vi "主界面.vi"() -> ()   [LabVIEW 2010]
uses:
  全局量/全局_配置.vi
  全局量/试验配置信息.vi
  全局量/自动测试结果.vi
panel:
  in  "?":enum32{"测试类型 1", "测试类型 2"}(tab)
  in  "单选_数字量输入":bool
  in  "单选_数字量输出":bool
  in  "单选_DSP输入":bool
  in  "单选_CAN检测":bool
  in  "单选_LAN检测":bool
  in  "单选_R232检测":bool
  in  "btn_数字输出":bool
  in  "btn_DSP输入":bool
  in  "btn_CAN总线":bool
  in  "btn_LAN总线":bool
  in  "btn_R232总线":bool
  in  "btn_开始检测":bool
  in  "btn_数字输入":bool
  in  "btn_R485总线":bool
  out "进度":u8(slide) scale=0.0..100.0
  in  "单选_R485检测":bool
  in  "单选_AD输入":bool
  out "数字量输入检测":bool
  out "数字量输出检测":bool
  out "模拟量DSP输入检测":bool
  out "模拟量AD输入检测":bool
  out "CAN总线检测":bool
  out "LAN总线检测":bool
  out "RS232总线检测":bool
  out "RS485总线检测":bool
  in  "函数类型 4":bool
  in  "通道及参数配置":bool
  in  "函数类型 2":bool
  in  "函数类型 3":bool
  in  "函数类型 1":bool
  in  "进度每次增加数":dbl
  in  "电路板类型":T1(ring)
  in  "btn_二维码识别":bool
  out "退出？":bool
  in  "btn_退出":bool
  out "时间标识":timestamp format="%<%H:%M:%S>T"
  in  "btn_报告管理":bool
  in  "btn_生成报表":bool
  in  "btn_保存结果":bool
  in  "str_测试地点":string
  in  "str_测试人员":string
  in  "str_测试编号":string
  in  "str_报告编号":string
  out "检测信息":string[][](table)
  in  "btn_控制板配置":bool
  # "TNB-S600KZ型控制板自动化检测装置"
  # "测试报告信息"
  # "板 卡 试  验  信  息"
  # "试验报告编号："
  # "测试板卡编号："
  # "板卡类型："
  # "测试人员："
  # "测试地点："
  # "系统时间:"
  # "自动检测"
  # "分步检测"
  # "检\n测\n项\n目"
  # "检测进度"
  # "配置选项"
  # "分步检测"
  # "检\n测\n项\n目"
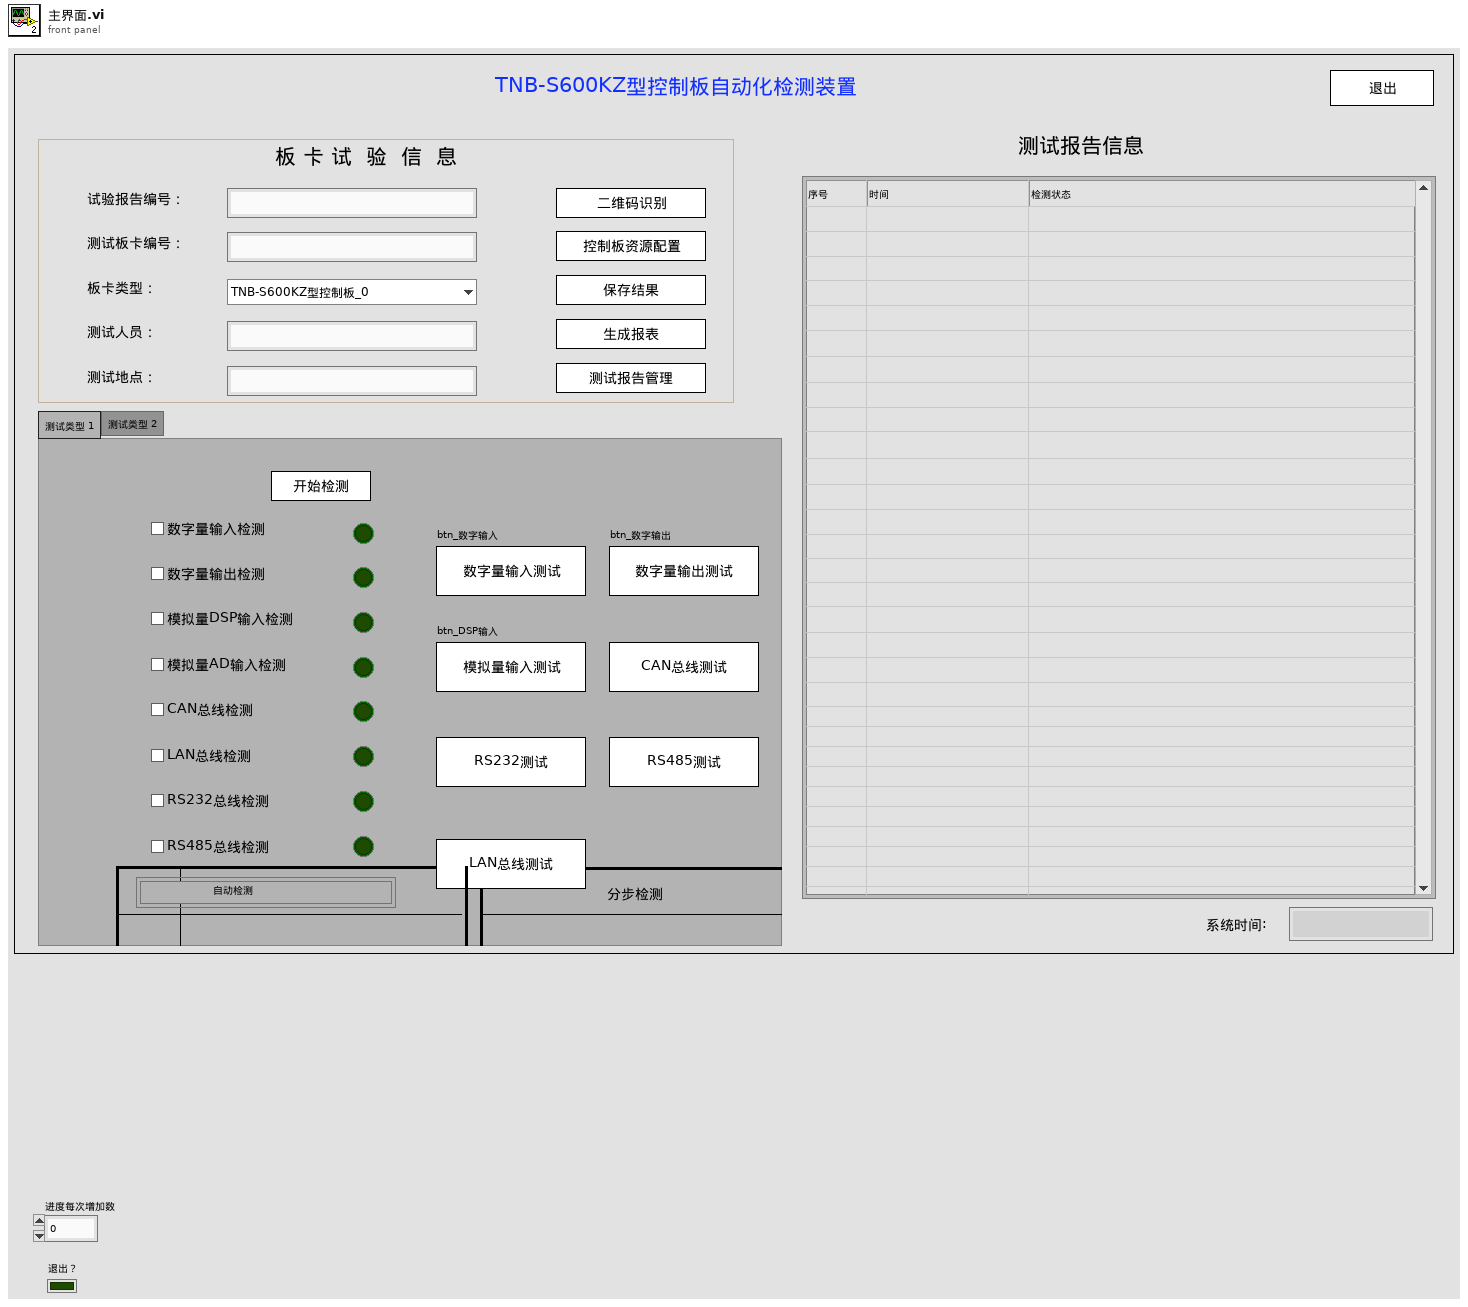
[diagram p1: front panel]
types:
  T1 = enum16{"TNB-S600KZ型控制板_0", "TNB-S600KZ型控制板_1", "TNB-S600KZ型控制板_2"}
  T2 = cluster{"数字量输入信号路数":u32, "数字量输出信号路数":u32, "DSP模拟量输入信号路数":u32, "DSP模拟量输入信号幅值":u32, "AD模拟量输入信号路数":u32, "AD模拟量输入信号幅值":u32, "RS232端口":u32, "RS232通信路数":u32, "RS232波特率":u32, "RS485端口":u32, "RS485通信路数":u32, "RS485波特率":u32, "CAN通信端口":string, "CAN波特率":u32, "以太网选择?":bool, "控制板IP":string, "以太网端口":u32}
  T3 = cluster{"str_报告编号":string, "str_测试板卡编号":string, "str_测试人员":string, "str_测试地点":string, "str_测试板卡类型":string}
  T4 = cluster{"str_报告编号":string, "str_测试编号":string, "str_测试人员":string, "str_测试地点":string, string}
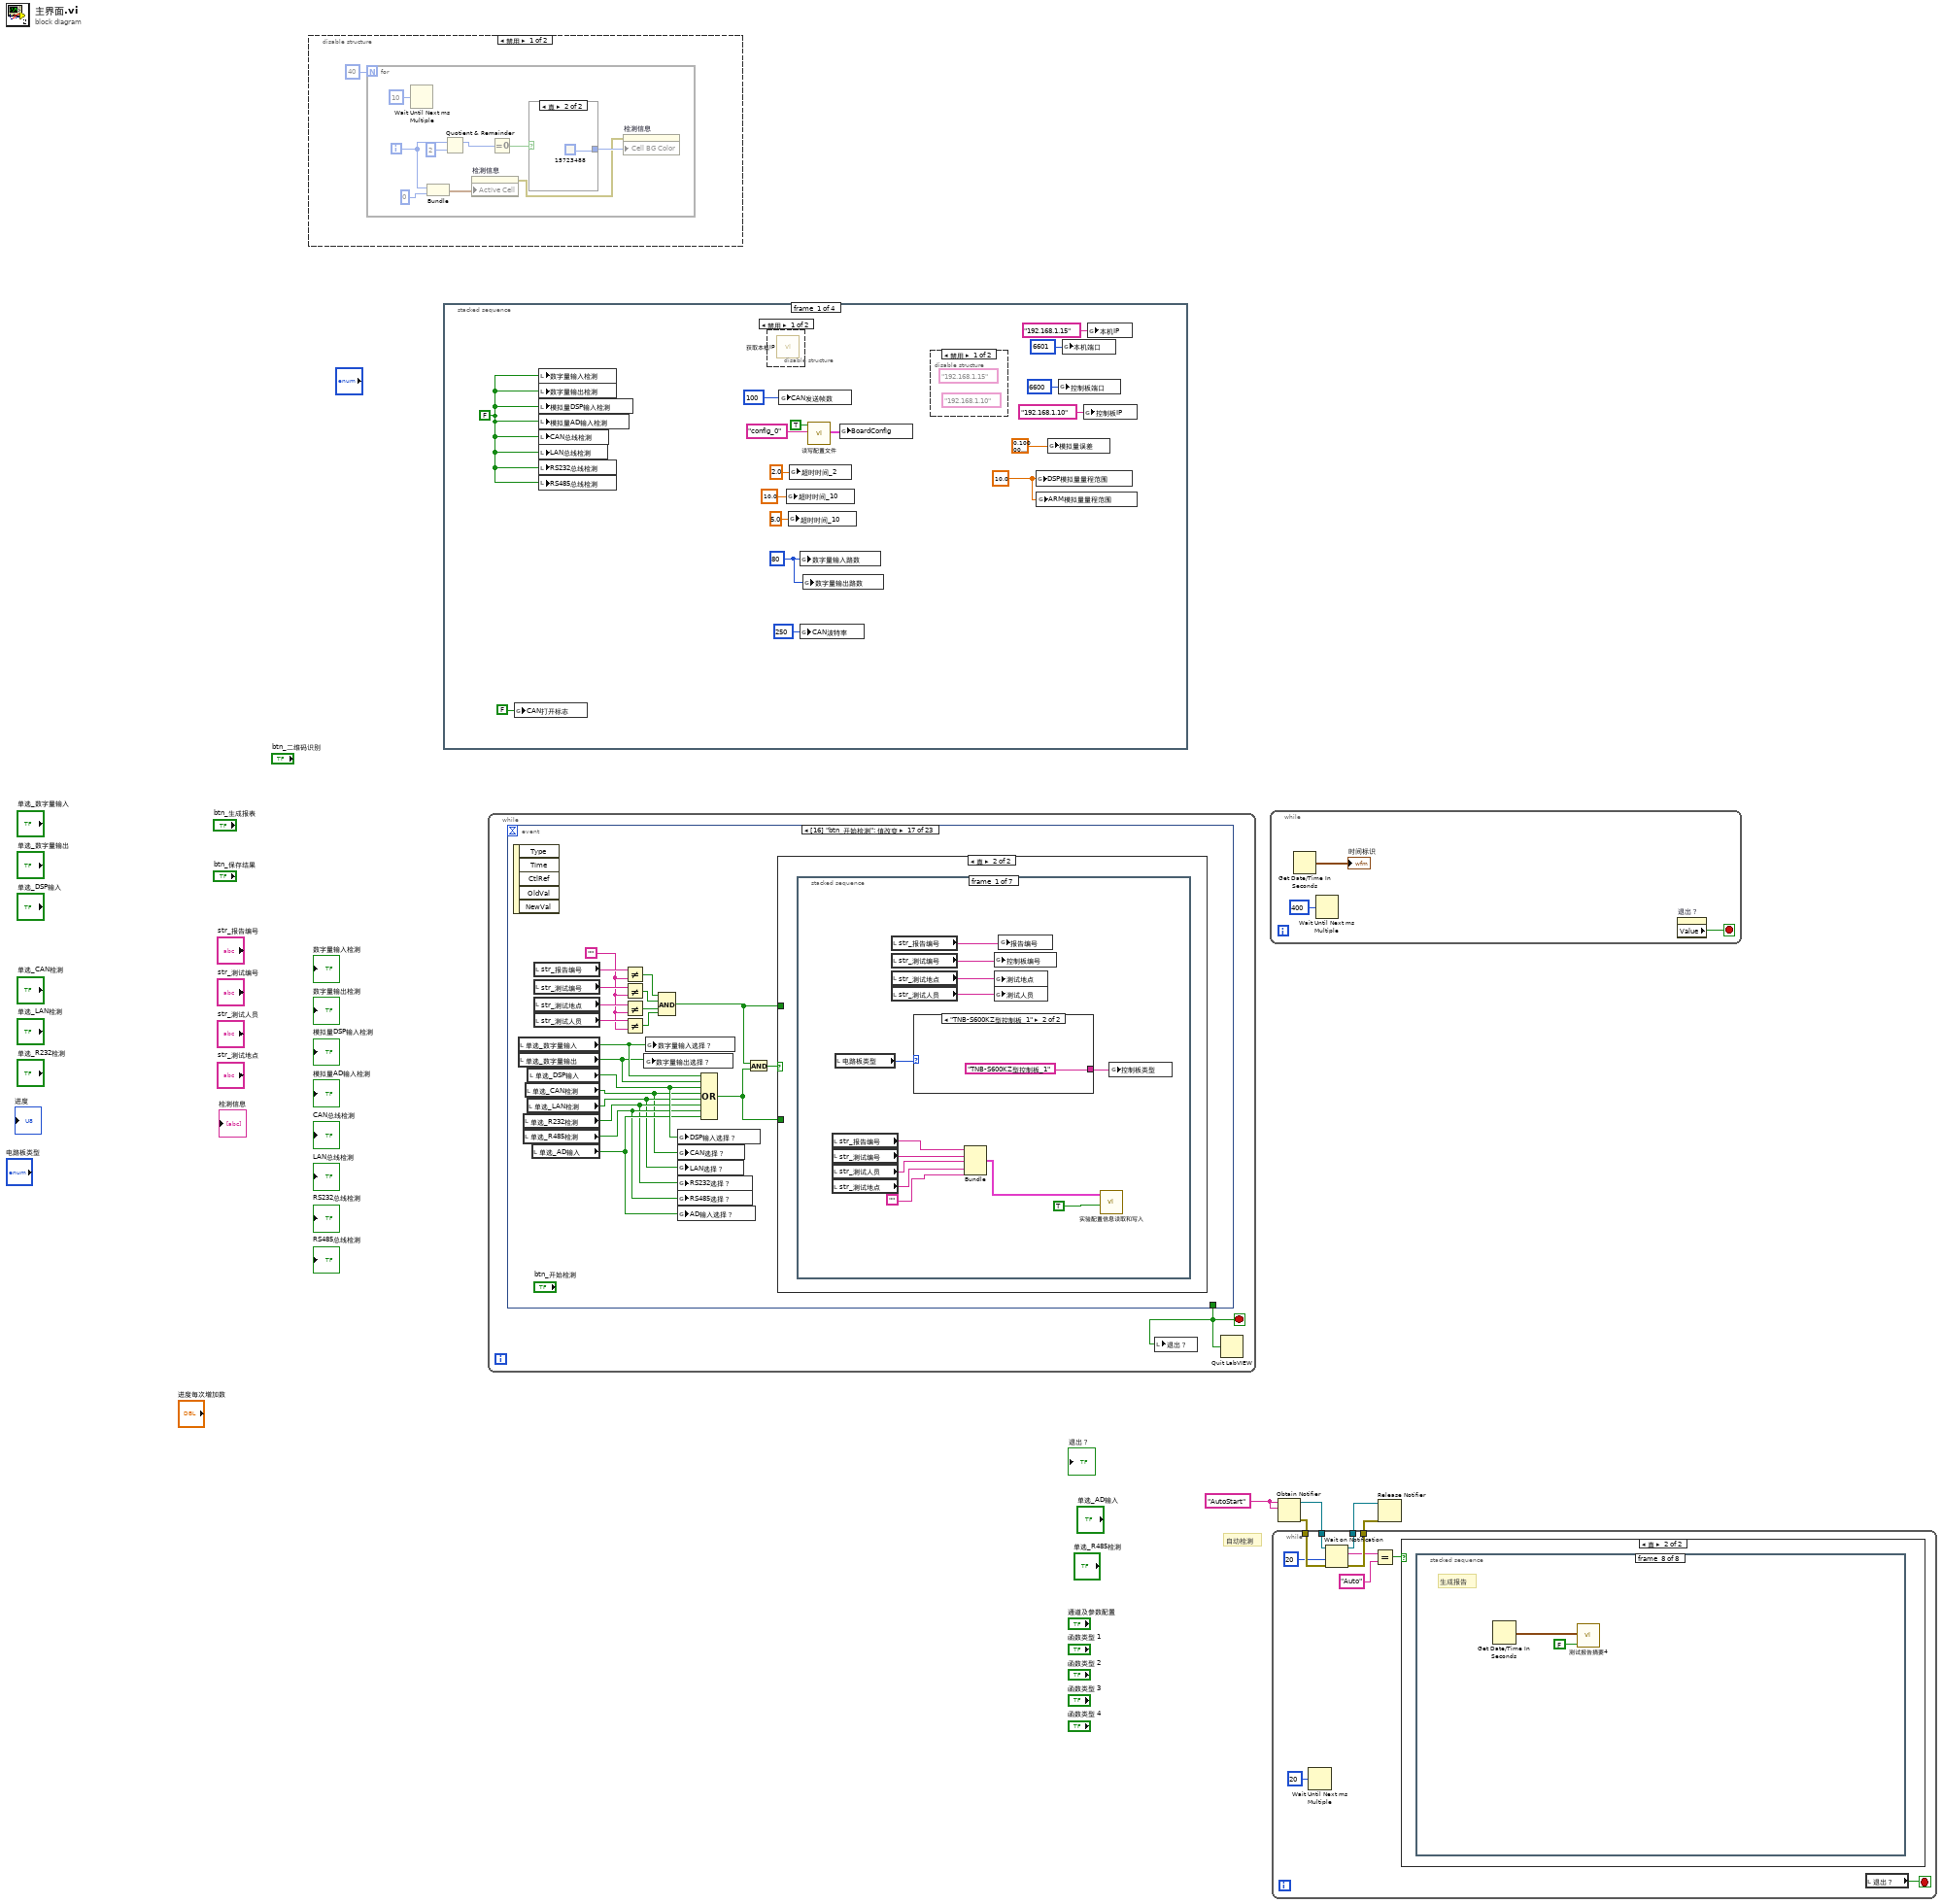
[diagram p0: block diagram]
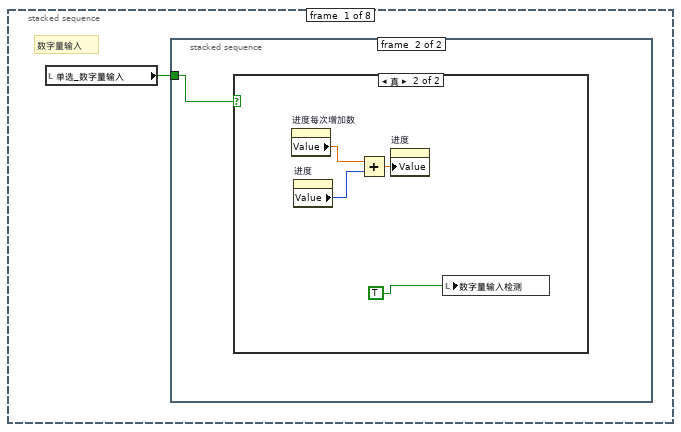
[diagram p3: hidden frame]
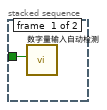
[diagram p4: hidden frame]
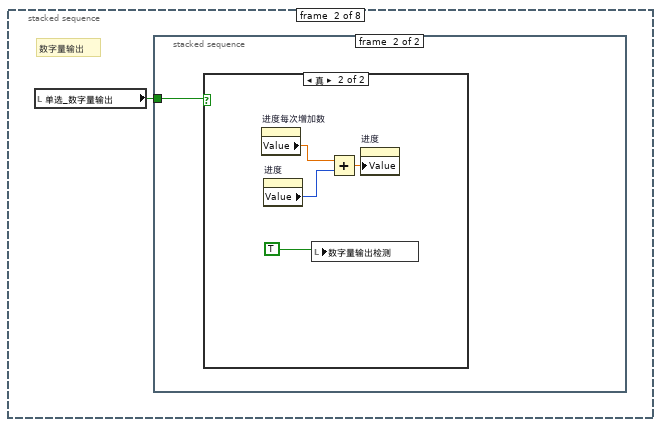
[diagram p6: hidden frame]
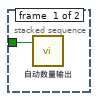
[diagram p7: hidden frame]
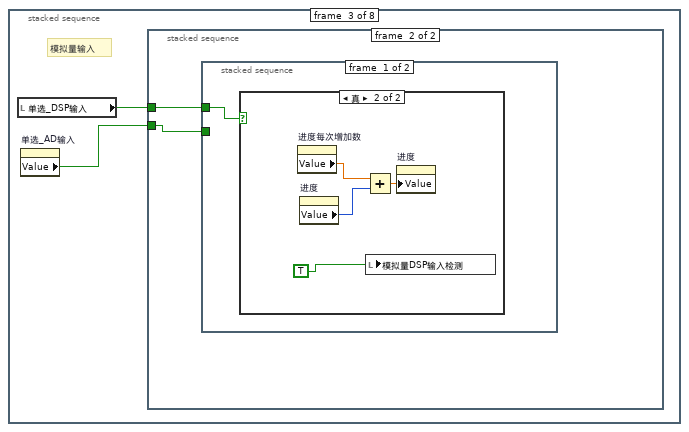
[diagram p9: hidden frame]
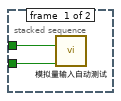
[diagram p10: hidden frame]
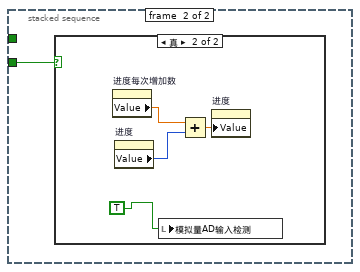
[diagram p12: hidden frame]
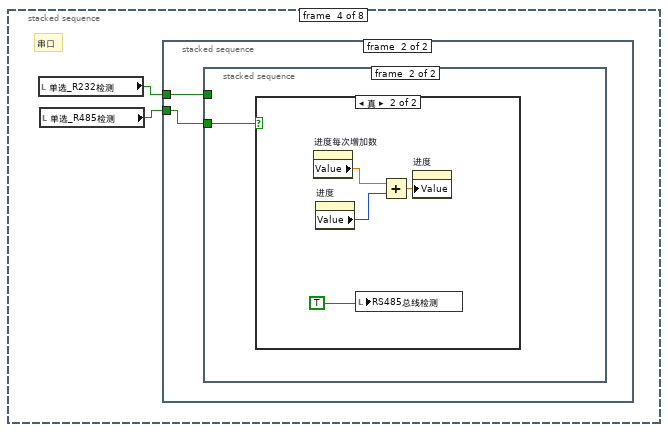
[diagram p14: hidden frame]
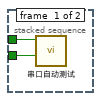
[diagram p15: hidden frame]
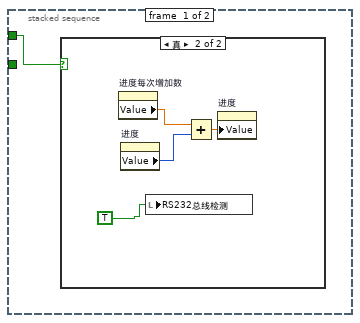
[diagram p16: hidden frame]
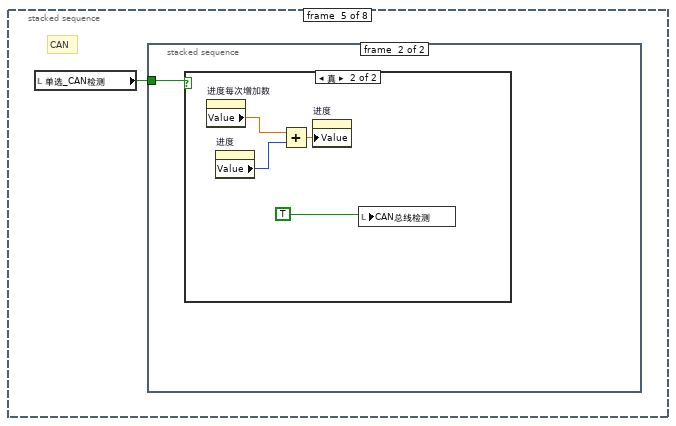
[diagram p19: hidden frame]
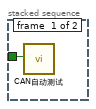
[diagram p20: hidden frame]
diagram:
  w5 = "AutoStart" ("名称（未命名）")
  # "自动检测"
  n1 = disable-structure shown="禁用" {
    frame Disabled {
      n2 = for {
        N: 40 -> [_]
        i -> [w10]
        n3 = Wait Until Next ms Multiple(millisecond multiple=u32 10 ("毫秒倍数")) -> ()  [unwired: 1 out]
        n4 = Bundle(w10, 0) -> (w11:cluster{i32, i32})  [unwired: 1 in]
        n5 = Quotient & Remainder(x=w10, y=2) -> (x-y*floor(x/y)=w8:i32)  [unwired: 1 out]
        n6 = property on="检测信息" class="Tbl (严格)"("Active Cell"=w11) -> (error out=w7:errorcluster)  [unwired: 2 in, 1 out]
        n7 = Equal To 0?(x=w8) -> (x = 0?=w15:bool)
        n8 = case shown="真" w15 {
          tunnel: [u32 16448250 u32 15723488] -> w14
          frame False {
          }
          frame True {
          }
        }
        n9 = property on="检测信息" class="Tbl (严格)"(error in=w7, "Cell BG Color"=w14) -> ()  [unwired: 1 in, 2 out]
      }
    }
    frame Enabled {
    }
  }
  n10 = stacked-sequence {
    frame #0 {
      w18 = FALSE
      w20 = 80 ("数字量输入路数")
      w21 = sgl 10.0 ("DSP模拟量量程范围")
      n11 = global write "全局_配置.vi" "CAN打开标志"(FALSE ("CAN打开标志")) -> ()
      n12 = local write "数字量输入检测"(w18) -> ()
      n13 = local write "数字量输出检测"(w18) -> ()
      n14 = local write "模拟量DSP输入检测"(w18) -> ()
      n15 = local write "模拟量AD输入检测"(w18) -> ()
      n16 = local write "CAN总线检测"(w18) -> ()
      n17 = local write "LAN总线检测"(w18) -> ()
      n18 = local write "RS232总线检测"(w18) -> ()
      n19 = local write "RS485总线检测"(w18) -> ()
      n20 = disable-structure shown="禁用" {
        frame Disabled {
          n21 = call "获取本机IP.vi"() -> ()  [unwired: 9 in, 3 out]
        }
        frame Enabled {
        }
      }
      n22 = global write "全局_配置.vi" "CAN发送帧数"(u32 100 ("CAN发送帧数")) -> ()
      n23 = global write "全局_配置.vi" "超时时间_10"(10.0 ("超时时间_102")) -> ()
      n24 = global write "全局_配置.vi" "超时时间_10"(5.0 ("超时时间_10")) -> ()
      n25 = global write "全局_配置.vi" "超时时间_2"(2.0 ("超时时间_2")) -> ()
      n26 = global write "全局_配置.vi" "数字量输入路数"(w20) -> ()
      n27 = global write "全局_配置.vi" "CAN波特率"(u16 250 ("CAN波特率")) -> ()
      n28 = global write "全局_配置.vi" "数字量输出路数"(w20) -> ()
      n29 = call "读写配置文件.vi"("文件名称"="config_0", "m_bRead"=TRUE) -> ("BoardConfig_output"=w32:T2)  [unwired: 9 in]
      n30 = global write "全局_配置.vi" "BoardConfig"(w32) -> ()
      n31 = disable-structure shown="禁用" {
        frame Disabled {
          (unwired) "192.168.1.15" ("本机IP")
          (unwired) "192.168.1.10" ("控制板IP")
        }
        frame Enabled {
        }
      }
      n32 = global write "全局_配置.vi" "DSP模拟量量程范围"(w21) -> ()
      n33 = global write "全局_配置.vi" "ARM模拟量量程范围"(w21) -> ()
      n34 = global write "全局_配置.vi" "模拟量误差"(sgl 0.1 ("模拟量误差")) -> ()
      n35 = global write "全局_配置.vi" "控制板端口"(u16 6600 ("控制板端口")) -> ()
      n36 = global write "全局_配置.vi" "本机端口"(u16 6601 ("本机端口")) -> ()
      n37 = global write "全局_配置.vi" "控制板IP"("192.168.1.10" ("控制板IP")) -> ()
      n38 = global write "全局_配置.vi" "本机IP"("192.168.1.15" ("本机IP")) -> ()
    }
    frame #1 {
      w41 = 16 ("维数大小")
      n39 = global write "试验配置信息.vi" "自测DO路数"(76 ("自测DO路数")) -> ()
      n40 = global write "试验配置信息.vi" "自测DI路数"(80 ("自测DI路数")) -> ()
      n41 = global write "试验配置信息.vi" "自测RS232路数"(2 ("自测RS232路数")) -> ()
      n42 = global write "试验配置信息.vi" "自测485路数"(1 ("自测485路数")) -> ()
      n43 = global write "试验配置信息.vi" "自测CAN路数"(4 ("自测CAN路数")) -> ()
      n44 = global write "试验配置信息.vi" "自测LAN路数"(1 ("自测LAN路数")) -> ()
      n45 = global write "试验配置信息.vi" "自测AI_DSP路数"(w41) -> ()
      n46 = global write "试验配置信息.vi" "自测AI_AD路数"(w41) -> ()
    }
    frame #2 {
      w58 = TRUE ("单选_数字量输入")
      # "自动测试"
      n47 = global write "自动测试结果.vi" "DI自动测试结果"(string[][] [["序号", "检测内容", "结果"]] ("自动测试结果")) -> ()
      n48 = local write "str_报告编号"("B001001000001" ("通知")) -> ()
      n49 = local write "str_测试地点"("1号实验室" ("str_测试地点")) -> ()
      n50 = global read "试验配置信息.vi" "自测AI_DSP路数"() -> (w54:i32)
      n51 = global read "试验配置信息.vi" "自测RS232路数"() -> (w43:i32)
      n52 = global read "试验配置信息.vi" "自测AI_AD路数"() -> (w53:i32)
      n53 = global read "试验配置信息.vi" "自测CAN路数"() -> (w49:i32)
      n54 = global read "试验配置信息.vi" "自测485路数"() -> (w46:i32)
      n55 = Initialize Array(TRUE ("元素"), w49) -> (w48:bool[])
      n56 = Initialize Array(TRUE ("元素"), w46) -> (w47:bool[])
      n57 = local write "单选_数字量输入"(w58) -> ()
      n58 = local write "单选_数字量输出"(w58) -> ()
      n59 = local write "单选_DSP输入"(w58) -> ()
      n60 = local write "单选_CAN检测"(w58) -> ()
      n61 = local write "单选_LAN检测"(w58) -> ()
      n62 = local write "单选_R232检测"(w58) -> ()
      n63 = local write "单选_R485检测"(w58) -> ()
      n64 = local write "单选_AD输入"(w58) -> ()
      n65 = Initialize Array(TRUE ("元素"), w54) -> (w59:bool[])
      n66 = Initialize Array(TRUE ("元素"), w43) -> (w42:bool[])
      n67 = Initialize Array(TRUE ("元素"), w53) -> (w51:bool[])
      n68 = global write "自动测试结果.vi" "Auto_RS485_R"(w47) -> ()
      n69 = global write "自动测试结果.vi" "Auto_RS232_R"(w42) -> ()
      n70 = global write "自动测试结果.vi" "Auto_CAN_R"(w48) -> ()
      n71 = global write "自动测试结果.vi" "Auto_DSP_R"(w59) -> ()
      n72 = global write "自动测试结果.vi" "Auto_AD_R"(w51) -> ()
      n73 = property on="进度" class="Slide (严格)"("Value"=u8 0 ("进度")) -> ()  [unwired: 2 in, 2 out]
      n74 = global write "试验配置信息.vi" "自测类数"(0 ("自动测试个数")) -> ()
    }
    frame #3 {
      n75 = call "实验配置信息读取和写入.vi"("读取写入"=FALSE) -> ("簇 2"=w67:T3)  [unwired: 10 in]
      n76 = Unbundle By Name(w67) -> ("str_报告编号"=w66:string, "str_测试板卡编号"=w65:string, "str_测试人员"=w64:string, "str_测试地点"=w63:string)  [unwired: 1 out]
      n77 = local write "str_报告编号"(w66) -> ()
      n78 = local write "str_测试编号"(w65) -> ()
      n79 = local write "str_测试人员"(w64) -> ()
      n80 = local write "str_测试地点"(w63) -> ()
    }
  }
  n81 = while {
    stop <- w69 stop-if-true
    n82 = event shown="[16] \"btn_开始检测\": 值改变" {
      selector: _ -> [_ _ _ _ _ _ _ _ _ _ _ _ _ _ _ _ _ _ _ _ _ _ _]
      dyn-events: _ -> [_ _ _ _ _ _ _ _ _ _ _ _ _ _ _ _ _ _ _ _ _ _ _]
      timeout: _ -> [_ _ _ _ _ _ _ _ _ _ _ _ _ _ _ _ _ _ _ _ _ _ _]
      tunnel: [_ w70 _ _ _ _ _ _ _ _ _ _ _ _ _ _ _ _ _ _ _ _ _] -> w69
      event Timeout {
        n83 = event-data() -> ()  [unwired: 1 in, 2 out]
      }
      event "btn_退出": Value Change {
        n84 = event-data() -> ()  [unwired: 1 in, 5 out]
        n85 = case shown="真" "btn_退出" {
          tunnel: [FALSE TRUE] -> w70
          frame False {
          }
          frame True {
          }
        }
      }
      event "btn_控制板配置": Value Change {
        n86 = event-data() -> ()  [unwired: 1 in, 5 out]
        n87 = call "控制板配置.vi"() -> ()  [unwired: 12 in]
      }
      event "btn_报告管理": Value Change {
        n88 = event-data() -> ()  [unwired: 1 in, 5 out]
        n89 = call "测试报告管理.vi"() -> ()  [unwired: 12 in]
      }
      event "单选_数字量输入": Value Change {
        n90 = event-data() -> ("NewVal"=w74:bool)  [unwired: 1 in, 4 out]
        n91 = local write "单选_数字量输入"(w74) -> ()
      }
      event "单选_数字量输出": Value Change {
        n92 = event-data() -> ("NewVal"=w75:bool)  [unwired: 1 in, 4 out]
        n93 = local write "单选_数字量输出"(w75) -> ()
      }
      event "单选_DSP输入": Value Change {
        n94 = event-data() -> ("NewVal"=w76:bool)  [unwired: 1 in, 4 out]
        n95 = local write "单选_DSP输入"(w76) -> ()
      }
      event "单选_CAN检测": Value Change {
        n96 = event-data() -> ("NewVal"=w77:bool)  [unwired: 1 in, 4 out]
        n97 = local write "单选_CAN检测"(w77) -> ()
      }
      event "单选_LAN检测": Value Change {
        n98 = event-data() -> ("NewVal"=w78:bool)  [unwired: 1 in, 4 out]
        n99 = local write "单选_LAN检测"(w78) -> ()
      }
      event "单选_R232检测": Value Change {
        n100 = event-data() -> ("NewVal"=w79:bool)  [unwired: 1 in, 4 out]
        n101 = local write "单选_R232检测"(w79) -> ()
      }
      event "btn_数字输入": Value Change {
        n102 = event-data() -> ()  [unwired: 1 in, 5 out]
        n103 = call "数字量输入配置.vi"() -> ()  [unwired: 12 in]
      }
      event "btn_数字输出": Value Change {
        n104 = event-data() -> ()  [unwired: 1 in, 5 out]
        n105 = call "数字量输出配置.vi"() -> ()  [unwired: 12 in]
      }
      event "btn_DSP输入": Value Change {
        n106 = event-data() -> ()  [unwired: 1 in, 5 out]
        n107 = call "32路模拟量输入.vi"() -> ()  [unwired: 12 in]
      }
      event "btn_CAN总线": Value Change {
        n108 = event-data() -> ()  [unwired: 1 in, 5 out]
        n109 = call "CAN总线测试.vi"() -> ()  [unwired: 12 in]
      }
      event "btn_LAN总线": Value Change {
        n110 = event-data() -> ()  [unwired: 1 in, 5 out]
        n111 = call "以太网测试界面.vi"() -> ()  [unwired: 12 in]
      }
      event "btn_R232总线": Value Change {
        n112 = event-data() -> ()  [unwired: 1 in, 5 out]
        n113 = call "RS232发送接收.vi"() -> ()  [unwired: 12 in]
      }
      event "btn_开始检测": Value Change {
        w95 = ""
        n114 = event-data() -> ()  [unwired: 1 in, 5 out]
        n115 = local read "单选_数字量输入"() -> (w87:bool)
        n116 = local read "单选_数字量输出"() -> (w86:bool)
        n117 = local read "单选_R232检测"() -> (w82:bool)
        n118 = local read "单选_R485检测"() -> (w83:bool)
        n119 = local read "单选_CAN检测"() -> (w80:bool)
        n120 = local read "单选_LAN检测"() -> (w81:bool)
        n121 = local read "单选_DSP输入"() -> (w85:bool)
        n122 = local read "单选_AD输入"() -> (w84:bool)
        n123 = local read "str_报告编号"() -> (w99:string)
        n124 = local read "str_测试编号"() -> (w98:string)
        n125 = local read "str_测试地点"() -> (w97:string)
        n126 = local read "str_测试人员"() -> (w96:string)
        n127 = Not Equal?(x=w99, y=w95) -> (x != y?=w94:bool)
        n128 = Not Equal?(x=w98, y=w95) -> (x != y?=w93:bool)
        n129 = Not Equal?(x=w97, y=w95) -> (x != y?=w92:bool)
        n130 = Not Equal?(x=w96, y=w95) -> (x != y?=w91:bool)
        n131 = global write "试验配置信息.vi" "数字量输出选择？"(w86) -> ()
        n132 = global write "试验配置信息.vi" "数字量输入选择？"(w87) -> ()
        n133 = Compound Arithmetic op=AND(w94, w93, w92, w91) -> (w89:bool)
        n134 = global write "试验配置信息.vi" "DSP输入选择？"(w85) -> ()
        n135 = global write "试验配置信息.vi" "CAN选择？"(w80) -> ()
        n136 = global write "试验配置信息.vi" "LAN选择？"(w81) -> ()
        n137 = global write "试验配置信息.vi" "RS232选择？"(w82) -> ()
        n138 = global write "试验配置信息.vi" "RS485选择？"(w83) -> ()
        n139 = global write "试验配置信息.vi" "AD输入选择？"(w84) -> ()
        n140 = Compound Arithmetic op=OR(w87, w86, w85, w80, w81, w82, w83, w84) -> (w88:bool)
        n141 = And(x=w89, y=w88) -> (x .and. y?=w90:bool)
        n142 = case shown="真" w90 {
          tunnel: w89 -> [w101 _]
          tunnel: w88 -> [w100 _]
          frame False {
            n143 = case shown="假" w100 {
              frame False {
                n144 = call "显示对话框信息2"() -> ()  [unwired: 10 in, 2 out]
              }
              frame True {
              }
            }
            n145 = case shown="假" w101 {
              frame False {
                n146 = call "显示对话框信息"() -> ()  [unwired: 10 in, 2 out]
              }
              frame True {
              }
            }
          }
          frame True {
            n147 = stacked-sequence {
              frame #0 {
                n148 = local read "str_报告编号"() -> (w107:string)
                n149 = local read "str_测试编号"() -> (w106:string)
                n150 = local read "str_测试人员"() -> (w105:string)
                n151 = local read "str_测试地点"() -> (w104:string)
                n152 = local read "电路板类型"() -> (w111:T1)
                n153 = local read "str_报告编号"() -> (w109:string)
                n154 = local read "str_测试编号"() -> (w110:string)
                n155 = local read "str_测试地点"() -> (w114:string)
                n156 = local read "str_测试人员"() -> (w113:string)
                n157 = case shown="\"TNB-S600KZ型控制板_1\"" w111 {
                  tunnel: ["TNB-S600KZ型控制板_0" "TNB-S600KZ型控制板_1"] -> w112
                  frame "TNB-S600KZ型控制板_0", Default {
                  }
                  frame "TNB-S600KZ型控制板_1" {
                  }
                }
                n158 = Bundle("str_报告编号"=w107, "str_测试编号"=w106, "str_测试人员"=w105, "str_测试地点"=w104, "") -> (w102:T4)  [unwired: 1 in]
                n159 = global write "试验配置信息.vi" "控制板编号"(w110) -> ()
                n160 = global write "试验配置信息.vi" "测试地点"(w114) -> ()
                n161 = global write "试验配置信息.vi" "测试人员"(w113) -> ()
                n162 = global write "试验配置信息.vi" "报告编号"(w109) -> ()
                n163 = call "实验配置信息读取和写入.vi"("读取写入"=TRUE, "簇"=w102) -> ()  [unwired: 9 in, 1 out]
                n164 = global write "试验配置信息.vi" "控制板类型"(w112) -> ()
              }
              frame #1 {
                n165 = local read "单选_数字量输入"() -> (w125:bool)
                n166 = local read "单选_数字量输出"() -> (w124:bool)
                n167 = local read "单选_R232检测"() -> (w119:bool)
                n168 = local read "单选_R485检测"() -> (w118:bool)
                n169 = local read "单选_CAN检测"() -> (w121:bool)
                n170 = local read "单选_LAN检测"() -> (w120:bool)
                n171 = local read "单选_DSP输入"() -> (w123:bool)
                n172 = local read "单选_AD输入"() -> (w117:bool)
                n173 = property on="进度" class="Slide (严格)"("Value"=u8 0 ("进度")) -> ()  [unwired: 2 in, 2 out]
                n174 = Build Array(w125, w124, w123, w121, w120, w119, w118, w117) -> (w122:bool[])
                n175 = for {
                  tunnel: w122 -> [w127] mode=indexing
                  n176 = case shown="真" w127 {
                    frame False {
                    }
                    frame True {
                      n177 = global read "试验配置信息.vi" "自测类数"() -> (w129:i32)
                      n178 = Increment(x=w129) -> (x+1=w128:i32)
                      n179 = global write "试验配置信息.vi" "自测类数"(w128) -> ()
                    }
                  }
                }
              }
              frame #2 {
                n180 = global read "试验配置信息.vi" "数字量输出选择？"() -> (w136:bool)
                n181 = global read "试验配置信息.vi" "数字量输入选择？"() -> (w137:bool)
                n182 = global read "试验配置信息.vi" "AD输入选择？"() -> (w134:bool)
                n183 = global read "试验配置信息.vi" "DSP输入选择？"() -> (w135:bool)
                n184 = global read "试验配置信息.vi" "CAN选择？"() -> (w133:bool)
                n185 = global read "试验配置信息.vi" "RS232选择？"() -> (w131:bool)
                n186 = global read "试验配置信息.vi" "RS485选择？"() -> (w130:bool)
                n187 = global read "试验配置信息.vi" "LAN选择？"() -> (w132:bool)
                n188 = case shown="真" w137 {
                  tunnel: [0 w162] -> w146
                  frame False {
                  }
                  frame True {
                    n189 = global read "试验配置信息.vi" "自测DI路数"() -> (w162:i32)
                  }
                }
                n190 = case shown="真" w136 {
                  tunnel: [0 w160] -> w145
                  frame False {
                  }
                  frame True {
                    n191 = global read "试验配置信息.vi" "自测DO路数"() -> (w160:i32)
                  }
                }
                n192 = case shown="真" w134 {
                  tunnel: [0 w158] -> w144
                  frame False {
                  }
                  frame True {
                    n193 = global read "试验配置信息.vi" "自测AI_AD路数"() -> (w158:i32)
                  }
                }
                n194 = case shown="真" w135 {
                  tunnel: [0 w156] -> w143
                  frame False {
                  }
                  frame True {
                    n195 = global read "试验配置信息.vi" "自测AI_DSP路数"() -> (w156:i32)
                  }
                }
                n196 = case shown="真" w133 {
                  tunnel: [0 w154] -> w142
                  frame False {
                  }
                  frame True {
                    n197 = global read "试验配置信息.vi" "自测CAN路数"() -> (w154:i32)
                  }
                }
                n198 = case shown="真" w131 {
                  tunnel: [0 w152] -> w141
                  frame False {
                  }
                  frame True {
                    n199 = global read "试验配置信息.vi" "自测RS232路数"() -> (w152:i32)
                  }
                }
                n200 = case shown="真" w130 {
                  tunnel: [0 w150] -> w140
                  frame False {
                  }
                  frame True {
                    n201 = global read "试验配置信息.vi" "自测485路数"() -> (w150:i32)
                  }
                }
                n202 = case shown="真" w132 {
                  tunnel: [0 w148] -> w139
                  frame False {
                  }
                  frame True {
                    n203 = global read "试验配置信息.vi" "自测LAN路数"() -> (w148:i32)
                  }
                }
                n204 = Compound Arithmetic op=ADD(w146, w145, w144, w143, w142, w141, w140, w139) -> (w138:i32)
                n205 = global write "试验配置信息.vi" "自测项数"(w138) -> ()
              }
              frame #3 {
                w170 = string[][] [["序号", "检测内容", "测试结果"]] ("自动测试结果")
                n206 = global read "试验配置信息.vi" "自测AI_DSP路数"() -> (w164:i32)
                n207 = global read "试验配置信息.vi" "自测AI_AD路数"() -> (w166:i32)
                n208 = global write "自动测试结果.vi" "总线通信自测结果"(w170) -> ()
                n209 = global write "自动测试结果.vi" "DI自动测试结果"(w170) -> ()
                n210 = global write "自动测试结果.vi" "DO自动测试结果"(w170) -> ()
                n211 = Initialize Array(0.0 ("元素"), w164) -> (w163:dbl[])
                n212 = Initialize Array(0.0 ("元素"), w166) -> (w167:dbl[])
                n213 = global write "自动测试结果.vi" "AI自动测试结果"(string[][] [["序号", "检测内容", "最大误差(%)", "测试结果"]] ("自动测试结果")) -> ()
                n214 = global write "自动测试结果.vi" "Auto_DSP_max_WC"(w163) -> ()
                n215 = global write "自动测试结果.vi" "Auto_AD_max_WC"(w167) -> ()
              }
              frame #4 {
                w175 = 16 ("维数大小")
                n216 = global read "试验配置信息.vi" "自测AI_DSP路数"() -> (w182:i32)
                n217 = global read "试验配置信息.vi" "自测RS232路数"() -> (w193:i32)
                n218 = global read "试验配置信息.vi" "自测DI路数"() -> (w174:i32)
                n219 = global read "试验配置信息.vi" "自测AI_AD路数"() -> (w183:i32)
                n220 = global read "试验配置信息.vi" "自测CAN路数"() -> (w187:i32)
                n221 = global read "试验配置信息.vi" "自测485路数"() -> (w190:i32)
                n222 = Quotient & Remainder(x=w174, y=w175) -> (floor(x/y)=w176:i32)  [unwired: 1 out]
                n223 = Initialize Array(TRUE ("元素"), w187) -> (w188:bool[])
                n224 = Initialize Array(TRUE ("元素"), w190) -> (w189:bool[])
                n225 = Initialize Array(TRUE ("元素"), w182) -> (w181:bool[])
                n226 = Initialize Array(TRUE ("元素"), w193) -> (w194:bool[])
                n227 = Initialize Array(TRUE ("元素"), w183) -> (w185:bool[])
                n228 = Initialize Array(TRUE, w176, w175) -> (w173:bool[][])
                n229 = Initialize Array(TRUE, 5 ("维数大小"), 16 ("维数大小")) -> (w179:bool[][])
                n230 = global write "自动测试结果.vi" "Auto_RS485_R"(w189) -> ()
                n231 = global write "自动测试结果.vi" "Auto_RS232_R"(w194) -> ()
                n232 = global write "自动测试结果.vi" "Auto_CAN_R"(w188) -> ()
                n233 = global write "自动测试结果.vi" "Auto_DSP_R"(w181) -> ()
                n234 = global write "自动测试结果.vi" "Auto_AD_R"(w185) -> ()
                n235 = global write "自动测试结果.vi" "Auto_DI_R"(w173) -> ()
                n236 = global write "自动测试结果.vi" "Auto_DO_R"(w179) -> ()
              }
              frame #5 {
                w195 = ""
                n237 = global read "试验配置信息.vi" "自测类数"() -> (w202:i32)
                n238 = global read "试验配置信息.vi" "自测项数"() -> (w199:i32)
                n239 = global read "试验配置信息.vi" "自测类数"() -> (w200:i32)
                n240 = global write "自动测试结果.vi" "数字量输入概述"(w195) -> ()
                n241 = global write "自动测试结果.vi" "数字量输出概述"(w195) -> ()
                n242 = global write "自动测试结果.vi" "模拟量DSP概述"(w195) -> ()
                n243 = global write "自动测试结果.vi" "模拟量AD概述结果"(w195) -> ()
                n244 = global write "自动测试结果.vi" "串口RS232测试概述"(w195) -> ()
                n245 = global write "自动测试结果.vi" "串口RS485测试概述"(w195) -> ()
                n246 = global write "自动测试结果.vi" "CAN测试概述"(w195) -> ()
                n247 = global write "自动测试结果.vi" "CAN测试概述"(w195) -> ()
                n248 = global write "自动测试结果.vi" "以太网测试概述"(w195) -> ()
                n249 = Divide(x=100, y=w202) -> (x/y=w204:dbl)
                n250 = property on="进度每次增加数" class="DigNum (严格)"("Value"=w204) -> ()  [unwired: 2 in, 2 out]
                n251 = Format Into String(format string="本报告测试项目共%d类，测试项总计%d项，其中：" ("时间格式字符串(%c)"), w200, w199) -> (resulting string=w197:string)  [unwired: 2 in, 1 out]
                n252 = Concatenate Strings(w197, "\r") -> (w198:string)
                n253 = global write "自动测试结果.vi" "自测总概述"(w198) -> ()
              }
              frame #6 {
                w206 = "AutoStart" ("名称（未命名）")
                n254 = Obtain Notifier(name (unnamed)=w206, notification data type=w206) -> (notifier out=w205:refnum<notifier>)  [unwired: 2 in, 2 out]
                n255 = Send Notification(notification="Auto" ("通知"), notifier=w205) -> ()  [unwired: 1 in, 2 out]
              }
            }
          }
        }
      }
      event "btn_R485总线": Value Change {
        n256 = event-data() -> ()  [unwired: 1 in, 5 out]
        n257 = call "RS485发送接收.vi"() -> ()  [unwired: 12 in]
      }
      event "通道及参数配置": Value Change {
        n258 = event-data() -> ()  [unwired: 1 in, 5 out]
        n259 = disable-structure shown="禁用" {
          frame Disabled {
            n260 = call "通道配置模块.vi"() -> ()  [unwired: 12 in]
          }
          frame Enabled {
          }
        }
      }
      event "函数类型 1": Value Change {
        n261 = event-data() -> ()  [unwired: 1 in, 5 out]
        n262 = call "函数类型1测试.vi"() -> ()  [unwired: 12 in]
      }
      event "函数类型 2": Value Change {
        n263 = event-data() -> ()  [unwired: 1 in, 5 out]
        n264 = call "函数类型2测试.vi"() -> ()  [unwired: 12 in]
      }
      event "函数类型 3": Value Change {
        n265 = event-data() -> ()  [unwired: 1 in, 5 out]
        n266 = call "函数类型3测试.vi"() -> ()  [unwired: 12 in]
      }
      event "函数类型 4": Value Change {
        n267 = event-data() -> ()  [unwired: 1 in, 5 out]
        n268 = call "函数类型4测试.vi"() -> ()  [unwired: 12 in]
      }
    }
    n269 = local write "退出？"(w69) -> ()
    n270 = Quit LabVIEW(quit? (T)=w69) -> ()
  }
  n271 = while {
    stop <- w208 stop-if-true
    n272 = Get Date/Time In Seconds() -> (seconds since 1Jan1904=→"时间标识":timestamp)
    n273 = Wait Until Next ms Multiple(millisecond multiple=u32 400 ("毫秒倍数")) -> ()  [unwired: 1 out]
    n274 = property on="退出？" class="Bool (严格)"() -> ("Value"=w208:bool)  [unwired: 2 in, 2 out]
  }
  n275 = Obtain Notifier(name (unnamed)=w5, notification data type=w5) -> (notifier out=w4:refnum<notifier>, error out=w3:errorcluster)  [unwired: 2 in, 1 out]
  n276 = while {
    tunnel: w4 -> [w220]
    tunnel: w3 -> [w219]
    tunnel: [w218] -> w2
    tunnel: [w217] -> w1
    stop <- w212 stop-if-true
    n277 = Wait Until Next ms Multiple(millisecond multiple=u32 20 ("毫秒倍数")) -> ()  [unwired: 1 out]
    n278 = Wait on Notification(notifier=w220, timeout in ms (-1)=20 ("超时毫秒(-1)"), error in (no error)=w219) -> (notifier out=w218:refnum<notifier>, notification=w215:string, error out=w217:errorcluster)  [unwired: 1 in, 1 out]
    n279 = Equal?(x=w215, y="Auto" ("通知")) -> (x = y?=w214:bool)
    n280 = case shown="真" w214 {
      frame False {
      }
      frame True {
        n281 = stacked-sequence {
          frame #0 {
            # "数字量输入"
            n282 = local read "单选_数字量输入"() -> (w221:bool)
            n283 = stacked-sequence {
              tunnel: w221 -> [w222 w223]
              frame #0 {
                n284 = call "数字量输入自动检测.vi"("选择?"=w222) -> ()  [unwired: 11 in]
              }
              frame #1 {
                n285 = case shown="真" w223 {
                  frame False {
                  }
                  frame True {
                    n286 = property on="进度每次增加数" class="DigNum (严格)"() -> ("Value"=w227:dbl)  [unwired: 2 in, 2 out]
                    n287 = property on="进度" class="Slide (严格)"() -> ("Value"=w226:u8)  [unwired: 2 in, 2 out]
                    n288 = Add(x=w227, y=w226) -> (x+y=w225:dbl)
                    n289 = property on="进度" class="Slide (严格)"("Value"=w225) -> ()  [unwired: 2 in, 2 out]
                    n290 = local write "数字量输入检测"(TRUE) -> ()
                  }
                }
              }
            }
          }
          frame #1 {
            # "数字量输出"
            n291 = local read "单选_数字量输出"() -> (w228:bool)
            n292 = stacked-sequence {
              tunnel: w228 -> [w229 w230]
              frame #0 {
                n293 = call "自动数量输出.vi"("选择？"=w229) -> ()  [unwired: 11 in]
              }
              frame #1 {
                n294 = case shown="真" w230 {
                  frame False {
                  }
                  frame True {
                    n295 = property on="进度每次增加数" class="DigNum (严格)"() -> ("Value"=w234:dbl)  [unwired: 2 in, 2 out]
                    n296 = property on="进度" class="Slide (严格)"() -> ("Value"=w233:u8)  [unwired: 2 in, 2 out]
                    n297 = local write "数字量输出检测"(TRUE) -> ()
                    n298 = Add(x=w234, y=w233) -> (x+y=w232:dbl)
                    n299 = property on="进度" class="Slide (严格)"("Value"=w232) -> ()  [unwired: 2 in, 2 out]
                  }
                }
              }
            }
          }
          frame #2 {
            # "模拟量输入"
            n300 = local read "单选_DSP输入"() -> (w236:bool)
            n301 = property on="单选_AD输入" class="Bool (严格)"() -> ("Value"=w235:bool)  [unwired: 2 in, 2 out]
            n302 = stacked-sequence {
              tunnel: w236 -> [w238 w240]
              tunnel: w235 -> [w237 w239]
              frame #0 {
                n303 = call "模拟量输入自动测试.vi"("AD选择?"=w237, "DSP选择?"=w238) -> ()  [unwired: 10 in]
              }
              frame #1 {
                n304 = stacked-sequence {
                  tunnel: w240 -> [w241 _]
                  tunnel: w239 -> [_ w246]
                  frame #0 {
                    n305 = case shown="真" w241 {
                      frame False {
                      }
                      frame True {
                        n306 = property on="进度每次增加数" class="DigNum (严格)"() -> ("Value"=w245:dbl)  [unwired: 2 in, 2 out]
                        n307 = property on="进度" class="Slide (严格)"() -> ("Value"=w244:u8)  [unwired: 2 in, 2 out]
                        n308 = Add(x=w245, y=w244) -> (x+y=w243:dbl)
                        n309 = local write "模拟量DSP输入检测"(TRUE) -> ()
                        n310 = property on="进度" class="Slide (严格)"("Value"=w243) -> ()  [unwired: 2 in, 2 out]
                      }
                    }
                  }
                  frame #1 {
                    n311 = case shown="真" w246 {
                      frame False {
                      }
                      frame True {
                        n312 = property on="进度每次增加数" class="DigNum (严格)"() -> ("Value"=w250:dbl)  [unwired: 2 in, 2 out]
                        n313 = property on="进度" class="Slide (严格)"() -> ("Value"=w249:u8)  [unwired: 2 in, 2 out]
                        n314 = local write "模拟量AD输入检测"(TRUE) -> ()
                        n315 = Add(x=w250, y=w249) -> (x+y=w248:dbl)
                        n316 = property on="进度" class="Slide (严格)"("Value"=w248) -> ()  [unwired: 2 in, 2 out]
                      }
                    }
                  }
                }
              }
            }
          }
          frame #3 {
            # "串口"
            n317 = local read "单选_R232检测"() -> (w252:bool)
            n318 = local read "单选_R485检测"() -> (w251:bool)
            n319 = stacked-sequence {
              tunnel: w252 -> [w254 w256]
              tunnel: w251 -> [w253 w255]
              frame #0 {
                n320 = call "串口自动测试.vi"("RS485选择"=w253, "RS232选择"=w254) -> ()  [unwired: 10 in]
              }
              frame #1 {
                n321 = stacked-sequence {
                  tunnel: w256 -> [w257 _]
                  tunnel: w255 -> [_ w262]
                  frame #0 {
                    n322 = case shown="真" w257 {
                      frame False {
                      }
                      frame True {
                        n323 = property on="进度每次增加数" class="DigNum (严格)"() -> ("Value"=w261:dbl)  [unwired: 2 in, 2 out]
                        n324 = property on="进度" class="Slide (严格)"() -> ("Value"=w260:u8)  [unwired: 2 in, 2 out]
                        n325 = local write "RS232总线检测"(TRUE) -> ()
                        n326 = Add(x=w261, y=w260) -> (x+y=w259:dbl)
                        n327 = property on="进度" class="Slide (严格)"("Value"=w259) -> ()  [unwired: 2 in, 2 out]
                      }
                    }
                  }
                  frame #1 {
                    n328 = case shown="真" w262 {
                      frame False {
                      }
                      frame True {
                        n329 = property on="进度每次增加数" class="DigNum (严格)"() -> ("Value"=w266:dbl)  [unwired: 2 in, 2 out]
                        n330 = property on="进度" class="Slide (严格)"() -> ("Value"=w265:u8)  [unwired: 2 in, 2 out]
                        n331 = local write "RS485总线检测"(TRUE) -> ()
                        n332 = Add(x=w266, y=w265) -> (x+y=w264:dbl)
                        n333 = property on="进度" class="Slide (严格)"("Value"=w264) -> ()  [unwired: 2 in, 2 out]
                      }
                    }
                  }
                }
              }
            }
          }
          frame #4 {
            # "CAN"
            n334 = local read "单选_CAN检测"() -> (w267:bool)
            n335 = stacked-sequence {
              tunnel: w267 -> [w268 w269]
              frame #0 {
                n336 = call "CAN自动测试.vi"("选择?"=w268) -> ()  [unwired: 11 in]
              }
              frame #1 {
                n337 = case shown="真" w269 {
                  frame False {
                  }
                  frame True {
                    n338 = property on="进度每次增加数" class="DigNum (严格)"() -> ("Value"=w273:dbl)  [unwired: 2 in, 2 out]
                    n339 = property on="进度" class="Slide (严格)"() -> ("Value"=w272:u8)  [unwired: 2 in, 2 out]
                    n340 = Add(x=w273, y=w272) -> (x+y=w271:dbl)
                    n341 = property on="进度" class="Slide (严格)"("Value"=w271) -> ()  [unwired: 2 in, 2 out]
                    n342 = local write "CAN总线检测"(TRUE) -> ()
                  }
                }
              }
            }
          }
          frame #5 {
            # "以太网"
            n343 = local read "单选_LAN检测"() -> (w274:bool)
            n344 = stacked-sequence {
              tunnel: w274 -> [w275 w276]
              frame #0 {
                n345 = call "以太网自动测试.vi"("选择?"=w275) -> ()  [unwired: 11 in]
              }
              frame #1 {
                n346 = case shown="真" w276 {
                  frame False {
                  }
                  frame True {
                    n347 = property on="进度每次增加数" class="DigNum (严格)"() -> ("Value"=w280:dbl)  [unwired: 2 in, 2 out]
                    n348 = property on="进度" class="Slide (严格)"() -> ("Value"=w279:u8)  [unwired: 2 in, 2 out]
                    n349 = Add(x=w280, y=w279) -> (x+y=w278:dbl)
                    n350 = local write "LAN总线检测"(TRUE) -> ()
                    n351 = property on="进度" class="Slide (严格)"("Value"=w278) -> ()  [unwired: 2 in, 2 out]
                  }
                }
              }
            }
          }
          frame #6 {
            # "统计合格率"
            n352 = call "统计合格率.vi"() -> ()  [unwired: 12 in]
          }
          frame #7 {
            # "生成报告"
            n353 = Get Date/Time In Seconds() -> (seconds since 1Jan1904=w282:timestamp)
            n354 = call "测试报告摘要4.vi"("打印?"=FALSE, "试验时间"=w282) -> ()  [unwired: 10 in]
          }
        }
      }
    }
    n355 = local read "退出？"() -> (w212:bool)
  }
  n356 = Release Notifier(notifier=w2, error in (no error)=w1) -> ()  [unwired: 1 in, 3 out]
